vi "add_one_command_codes.vi"(2 "error in":errorcluster, 3 "Single Command Spec":T1, 4 "VI Ref In":refnum<vi>) -> (0 "error out":errorcluster, 1 "VI Ref Out":refnum<vi>)   [LabVIEW 2018]
uses:
  TypeDefinitions/single_cmd_spec.ctl
  TypeDefinitions/single_control_spec.ctl
  TypeDefinitions/control_data_type.ctl
  TypeDefinitions/control_class.ctl
  TypeDefinitions/ring_string_and_value.ctl
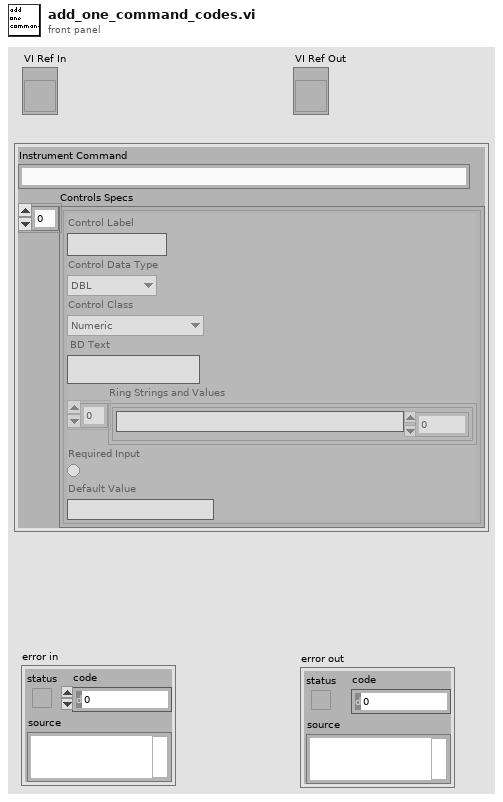
[diagram p1: front panel]
types:
  T1 = typedef "single_cmd_spec.ctl" = cluster{"Instrument Command":string, "Controls Specs":T2[]}
  T2 = typedef "single_control_spec.ctl" = cluster{"Control Label":string, "Control Data Type":T3, "Control Class":T4, "BD Text":string, "Ring Strings and Values":T5[], "Required Input":bool, "Default Value":string}
  T3 = typedef "control_data_type.ctl" = enum16{"DBL", "I32", "Boolean", "String", "U16", "U32", "EXT", "SGL", "I16", "U8", "I8", "I64", "U64", "Waveform", "Reference", "Variant", "Cluster"}
  T4 = typedef "control_class.ctl" = enum16{"Numeric", "Vertical Slide Switch", "Text Ring", "String", "Array", "VISAName", "WaveformGraph", "Cluster"}
  T5 = typedef "ring_string_and_value.ctl" = cluster{"String":string, "Value":dbl}
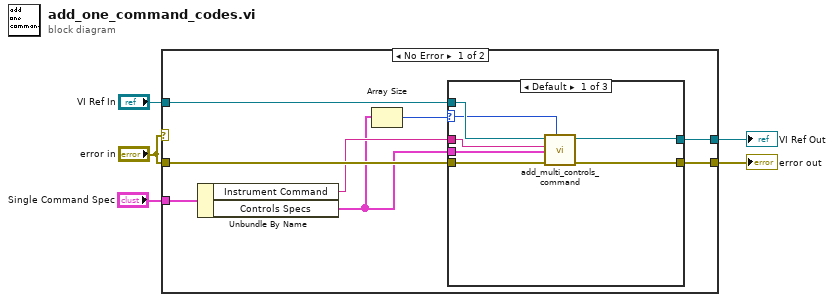
[diagram p0: block diagram]
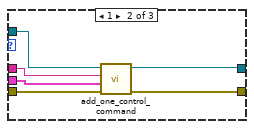
[diagram p2: hidden frame]
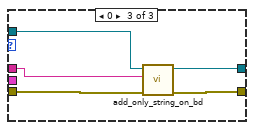
[diagram p3: hidden frame]
diagram:
  n1 = case shown="No Error" "error in" {
    selector: "error in" -> [_ w33]
    tunnel: [w13 w33] -> w5
    tunnel: "error in" -> [w12 _]
    tunnel: [w9 w32] -> w4
    tunnel: "Single Command Spec" -> [w7 _]
    tunnel: "VI Ref In" -> [w6 w32]
    frame No Error {
      n2 = Unbundle By Name(w7) -> ("Instrument Command"=w10:string, "Controls Specs"=w8:T2[])
      n3 = Array Size(array=w8) -> (size(s)=w11:i32)
      n4 = case shown="Default" w11 {
        selector: w11 -> [w17 _ _]
        tunnel: w8 -> [w20 w26 _]
        tunnel: w6 -> [w19 w25 w31]
        tunnel: [w14 w24 w30] -> w9
        tunnel: w10 -> [w18 w23 w28]
        tunnel: w12 -> [w16 w22 w29]
        tunnel: [w15 w21 w27] -> w13
        frame Default {
          n5 = call "add_multi_controls_command.vi"("Numeric"=w17, "error in"=w16, "Controls Specs"=w20, "Instrument Command"=w18, "VI Ref In"=w19) -> ("error out"=w15:errorcluster, "VI Ref Out"=w14:refnum<vi>)  [unwired: 5 out]
        }
        frame 1 {
          n6 = call "add_one_control_command.vi"("error in"=w22, "Controls Specs"=w26, "Instrument Command"=w23, "VI Ref In"=w25) -> ("error out"=w21:errorcluster, "VI Ref Out"=w24:refnum<vi>)  [unwired: 6 out]
        }
        frame 0 {
          n7 = call "add_only_string_on_bd.vi"("error in"=w29, "Instrument Command"=w28, "VI Ref In"=w31) -> ("error out"=w27:errorcluster, "VI Ref Out"=w30:refnum<vi>)  [unwired: 7 out]
        }
      }
    }
    frame Error {
    }
  }
  "error out" <- w5
  "VI Ref Out" <- w4
